vi "Measure vs B2Dv5beta_2.vi"() -> ()   [LabVIEW 2009]
doc: "This VI is an example operator panel.\n\nThe VI contains a table for the field values that may be configured manually, or loaded by checking the \"Prompt for File\" box. The data file should contain 3 columns of data, with each column delimited by a tab character.\n\nBefore the VI is executed, set the desired field units and coordinate system. Once the VI is started, follow the directions in the STATUS indicator to operate. Once a field value is achieved, it will be held indefinitely with no user intervention.\n\nThe present field is displayed in the selected units and coordinate system. The present field is queried once per second.\n\nIf a field point is specified that is outside the limits for the magnet, the VI will abort execution."
uses:
  <vilib>/Utility/file.llb/Read From Spreadsheet File (DBL).vi
panel:
  in  "AH":bool=TRUE
  in  "GPIB HP 2":string="13"
  in  "Z-Axis ramp?":bool=TRUE
  in  "Y- Axis ramp?":bool=TRUE
  out "Ist-Länge":dbl=0.009099999999997922
  out "z input":dbl=-3.5494
  out "y input":dbl=-3.5137
  out "Soll-Länge":dbl=4.994429702178218
  in  "FieldRange":dbl=1.0
  in  "Change\nPID\n(DetermineSIMPID.vi)":bool
  in  "X Axis":enum16{"B", "phi"}(ring)=enum."phi"
  in  "Y Axis":T1(ring)=enum."HP (V)"
  out "measured data":dbl[][](array[numeric])
  out "XY Graph":T2(graph)
  in  "Notes:":string="Datum: 5.09.11, Uhrzeit: 17:00, T1.5K, PID LOOP: P 0.5 I 200 D off , PID Dämpfung: P -0.5 D4.4E-5 , Laser 25°, 20mA, AOM 10mA, Sweep 0.09T/min, Winkelsweep 45-225° bei 0.5 T, VectorsM1.txt,  Winkelschritt 2°, mit ManualRamp" caption="Notizen:"
  out "Messfile Refnum":refnum<file>
  in  "Measurement File":path=path "D:/UserData/Matthias/Messungen/STO_LAOR103/110905/110905_R103_0.5T_winkelsweep_M1.txt"
  in  "Sample name:":string="R103"
  in  "HP 1":bool=TRUE
  in  "GPIB HP":string="14"
  in  "HP 2":bool=TRUE
  in  "LI 3":bool
  in  "GPIB L 3":string="8"
  in  "LI 2":bool
  in  "GPIB L 2":string="8"
  in  "LI 1":bool
  in  "GPIB L 1":string="8"
  out "Number of lines":i32=91
  out "Ramp Rate along Vector (T/min)":dbl=0.09 format="%.3f"
  out "Current Ramp Rate Z (T/min)":dbl=0.06396045575747722 format="%.3f"
  out "Current Ramp Rate Y (T/min)":dbl=0.06331713906436233 format="%.3f"
  in  "User defined Ramp Rate (T/min)":bool=TRUE
  in  "User defined Ramp Rate (T/min)":dbl=0.09 format="%.3f"
  in  "Z-Axis Communications Config":T3={"GPIB address"=22, "GPIB bus"=1, "connection ID"=refnum, "IP"="111.111.111.1", "Active Comm Interface"=0, "Serial Port"="", "Programmer Type"=0} {"Programmer Type" items=["Model 430", "Model 420"]; "Active Comm Interface" items=["TCP/IP (Model 430 Only)", "RS232", "IEEE488"]}
  in  "Max Ramp Rate - Y Axis (A/s)":dbl=0.055 format="%.3f"
  in  "Max Ramp Rate - Z Axis (A/s)":dbl=0.19 format="%.3f"
  in  "Magnitude Limit (kG)":dbl=45.1 format="%.3f"
  in  "Y-Axis Communications Config":T3={"GPIB address"=22, "GPIB bus"=1, "connection ID"=refnum, "IP"="111.111.111.2", "Active Comm Interface"=0, "Serial Port"="", "Programmer Type"=0} {"Programmer Type" items=["Model 430", "Model 420"]; "Active Comm Interface" items=["TCP/IP (Model 430 Only)", "RS232", "IEEE488"]}
  out "Cartesian Display (T)":T4={"Y-Axis Field (T)"=-8e-05, "Z-Axis Field (T)"=0.00027} {"Z-Axis Field (T)" format="%.3f"; "Y-Axis Field (T)" format="%.3f"}
  in  "Starting index":i32=92
  in  "Normal color":u32(colorbox)=11711154
  in  "Highlight color":u32(colorbox)=16711680
  in  "Prompt for File?":bool=TRUE
  out "Continue Execution?":bool=TRUE
  out "error out":T5
  in  "error in":T5
  out "STATUS":string="Zeroing vector."
  in  "Ramping Control":u16(ring)=4 items=["NEXT VECTOR", "RAMPING", "HOLDING", "PAUSE", "ZERO"]
  out "Cartesian Display (kG)":T6 {"Z-Axis Field (kG)" format="%.3f"; "Y-Axis Field (kG)" format="%.3f"}
  in  "Field Values":string[][](table)=[["0.5000", "45.0000"], ["0.5000", "47.0000"], ["0.5000", "49.0000"], ["0.5000", "51.0000"], ["0.5000", "53.0000"], ["0.5000", "55.0000"], ["0.5000", "57.0000"], ["0.5000", "59.0000"], ["0.5000", "61.0000"], ["0.5000", "63.0000"], ["0.5000", "65.0000"], ["0.5000", "67.0000"], ["0.5000", "69.0000"], ["0.5000", "71.0000"], ["0.5000", "73.0000"], ["0.5000", "75.0000"], ["0.5000", "77.0000"], ["0.5000", "79.0000"], ["0.5000", "81.0000"], ["0.5000", "83.0000"], ["0.5000", "85.0000"], ["0.5000", "87.0000"], ["0.5000", "89.0000"], ["0.5000", "91.0000"], ["0.5000", "93.0000"], ["0.5000", "95.0000"], ["0.5000", "97.0000"], ["0.5000", "99.0000"], ["0.5000", "101.0000"], ["0.5000", "103.0000"], ["0.5000", "105.0000"], ["0.5000", "107.0000"], ["0.5000", "109.0000"], ["0.5000", "111.0000"], ["0.5000", "113.0000"], ["0.5000", "115.0000"], ["0.5000", "117.0000"], ["0.5000", "119.0000"], ["0.5000", "121.0000"], ["0.5000", "123.0000"], ["0.5000", "125.0000"], ["0.5000", "127.0000"], ["0.5000", "129.0000"], ["0.5000", "131.0000"], ["0.5000", "133.0000"], ["0.5000", "135.0000"], ["0.5000", "137.0000"], ["0.5000", "139.0000"], ["0.5000", "141.0000"], ["0.5000", "143.0000"], ["0.5000", "145.0000"], ["0.5000", "147.0000"], ["0.5000", "149.0000"], ["0.5000", "151.0000"], ["0.5000", "153.0000"], ["0.5000", "155.0000"], ["0.5000", "157.0000"], ["0.5000", "159.0000"], ["0.5000", "161.0000"], ["0.5000", "163.0000"], ["0.5000", "165.0000"], ["0.5000", "167.0000"], ["0.5000", "169.0000"], ["0.5000", "171.0000"], ["0.5000", "173.0000"], ["0.5000", "175.0000"], ["0.5000", "177.0000"], ["0.5000", "179.0000"], ["0.5000", "181.0000"], ["0.5000", "183.0000"], ["0.5000", "185.0000"], ["0.5000", "187.0000"], ["0.5000", "189.0000"], ["0.5000", "191.0000"], ["0.5000", "193.0000"], ["0.5000", "195.0000"], ["0.5000", "197.0000"], ["0.5000", "199.0000"], ["0.5000", "201.0000"], ["0.5000", "203.0000"], ["0.5000", "205.0000"], ["0.5000", "207.0000"], ["0.5000", "209.0000"], ["0.5000", "211.0000"], ["0.5000", "213.0000"], ["0.5000", "215.0000"], ["0.5000", "217.0000"], ["0.5000", "219.0000"], ["0.5000", "221.0000"], ["0.5000", "223.0000"], ["0.5000", "225.0000"]]
  out "Switch Heaters":bool=TRUE
  out "Polar Display (T)":T7 {"Field Magnitude (T)" format="%.3f"; "q (degrees)" format="%.3f"}
  out "Polar Display (kG)":T8 {"Field Magnitude (kG)" format="%.3f"; "q (degrees)" format="%.3f"}
  in  "Coordinate System":u16(ring)=1 items=["Cartesian", "Polar"]
  in  "Magnetic Field Units":u16(ring)=1 items=["kG", "Tesla"]
  # "Vorsicht! Preliminary Measurement Program, watch field limits and pause the power supplies manually when stopping \nthe program!"
  # "Measurement Display"
  # "Measurement Settings"
  # "Magnet Settings"
  # "Max Ramp Rate z: 1.27 T/min\nMax Ramp Rate y: 0.17 T/min"
  # "Devices"
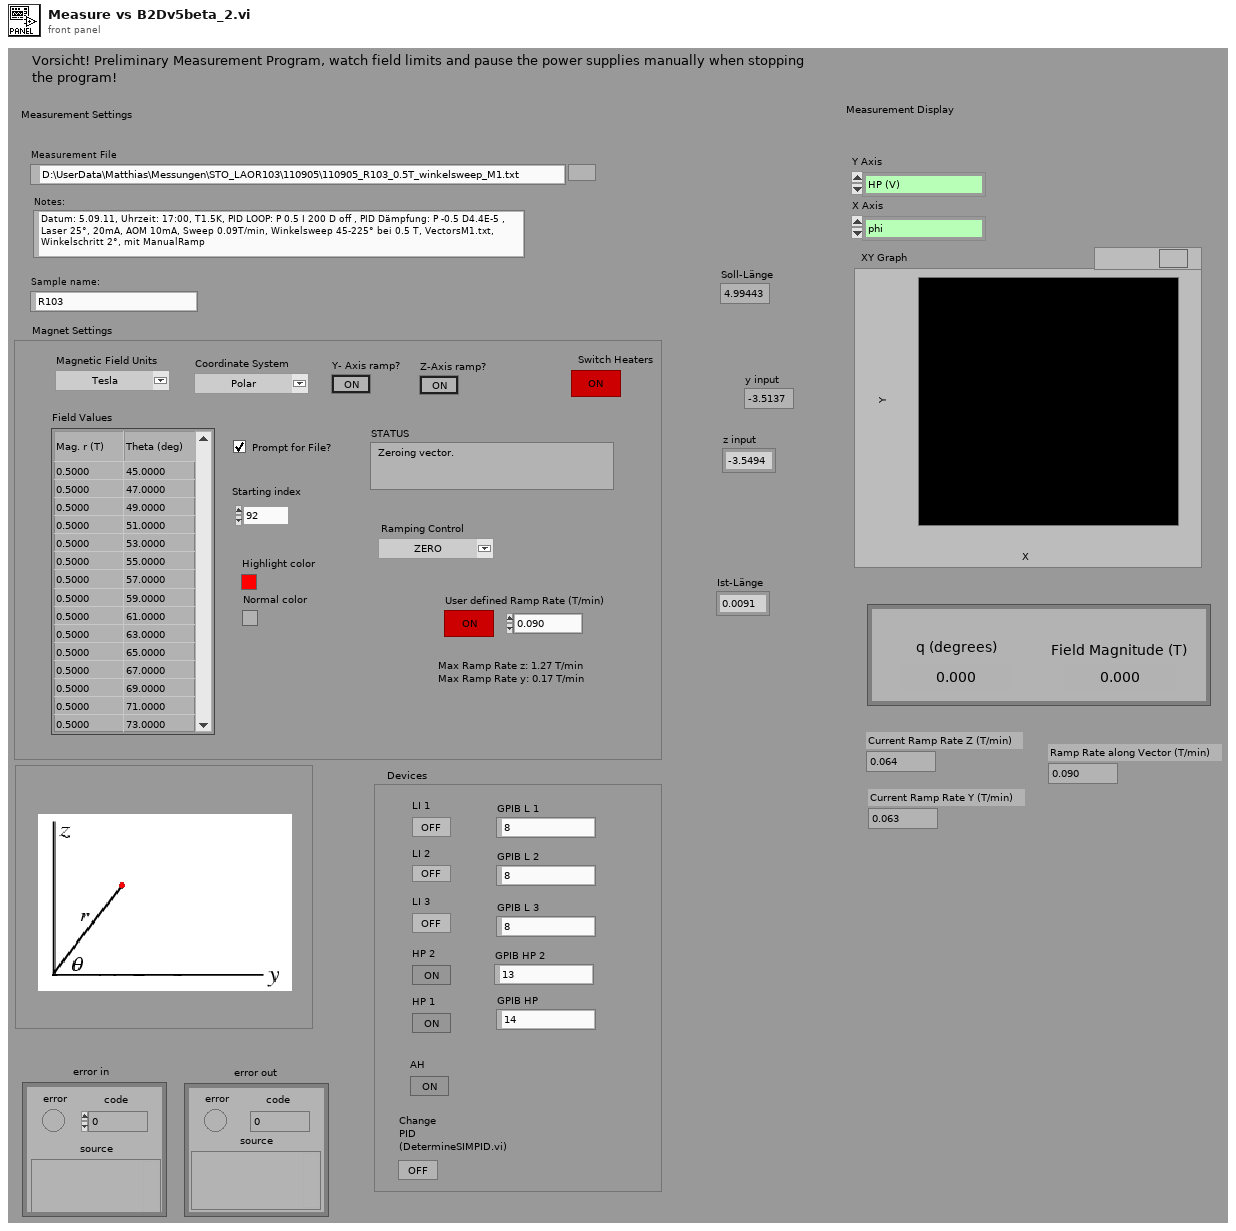
[diagram p1: front panel]
types:
  T1 = enum16{"B", "phi", "LI 1 Vx", "LI 1 phase", "LI 2 Vx", "LI 2 phase", "LI 3 Vx", "LI 3 phase", "LI 4 Vx", "LI 4 phase", "HP (V)"}
  T2 = cluster{"measured data":dbl[], "measured data":dbl[]}
  T3 = cluster{"GPIB address":i16, "GPIB bus":i16, "connection ID":refnum<k5>, "IP":string, "Active Comm Interface":u16, "Serial Port":refnum<visa-resource-name>, "Programmer Type":u16}
  T4 = cluster{"Y-Axis Field (T)":dbl, "Z-Axis Field (T)":dbl}
  T5 = cluster{"error":bool, "code":i32, "source":string}
  T6 = cluster{"Y-Axis Field (kG)":dbl, "Z-Axis Field (kG)":dbl}
  T7 = cluster{"q (degrees)":dbl, "Field Magnitude (T)":dbl}
  T8 = cluster{"q (degrees)":dbl, "Field Magnitude (kG)":dbl}
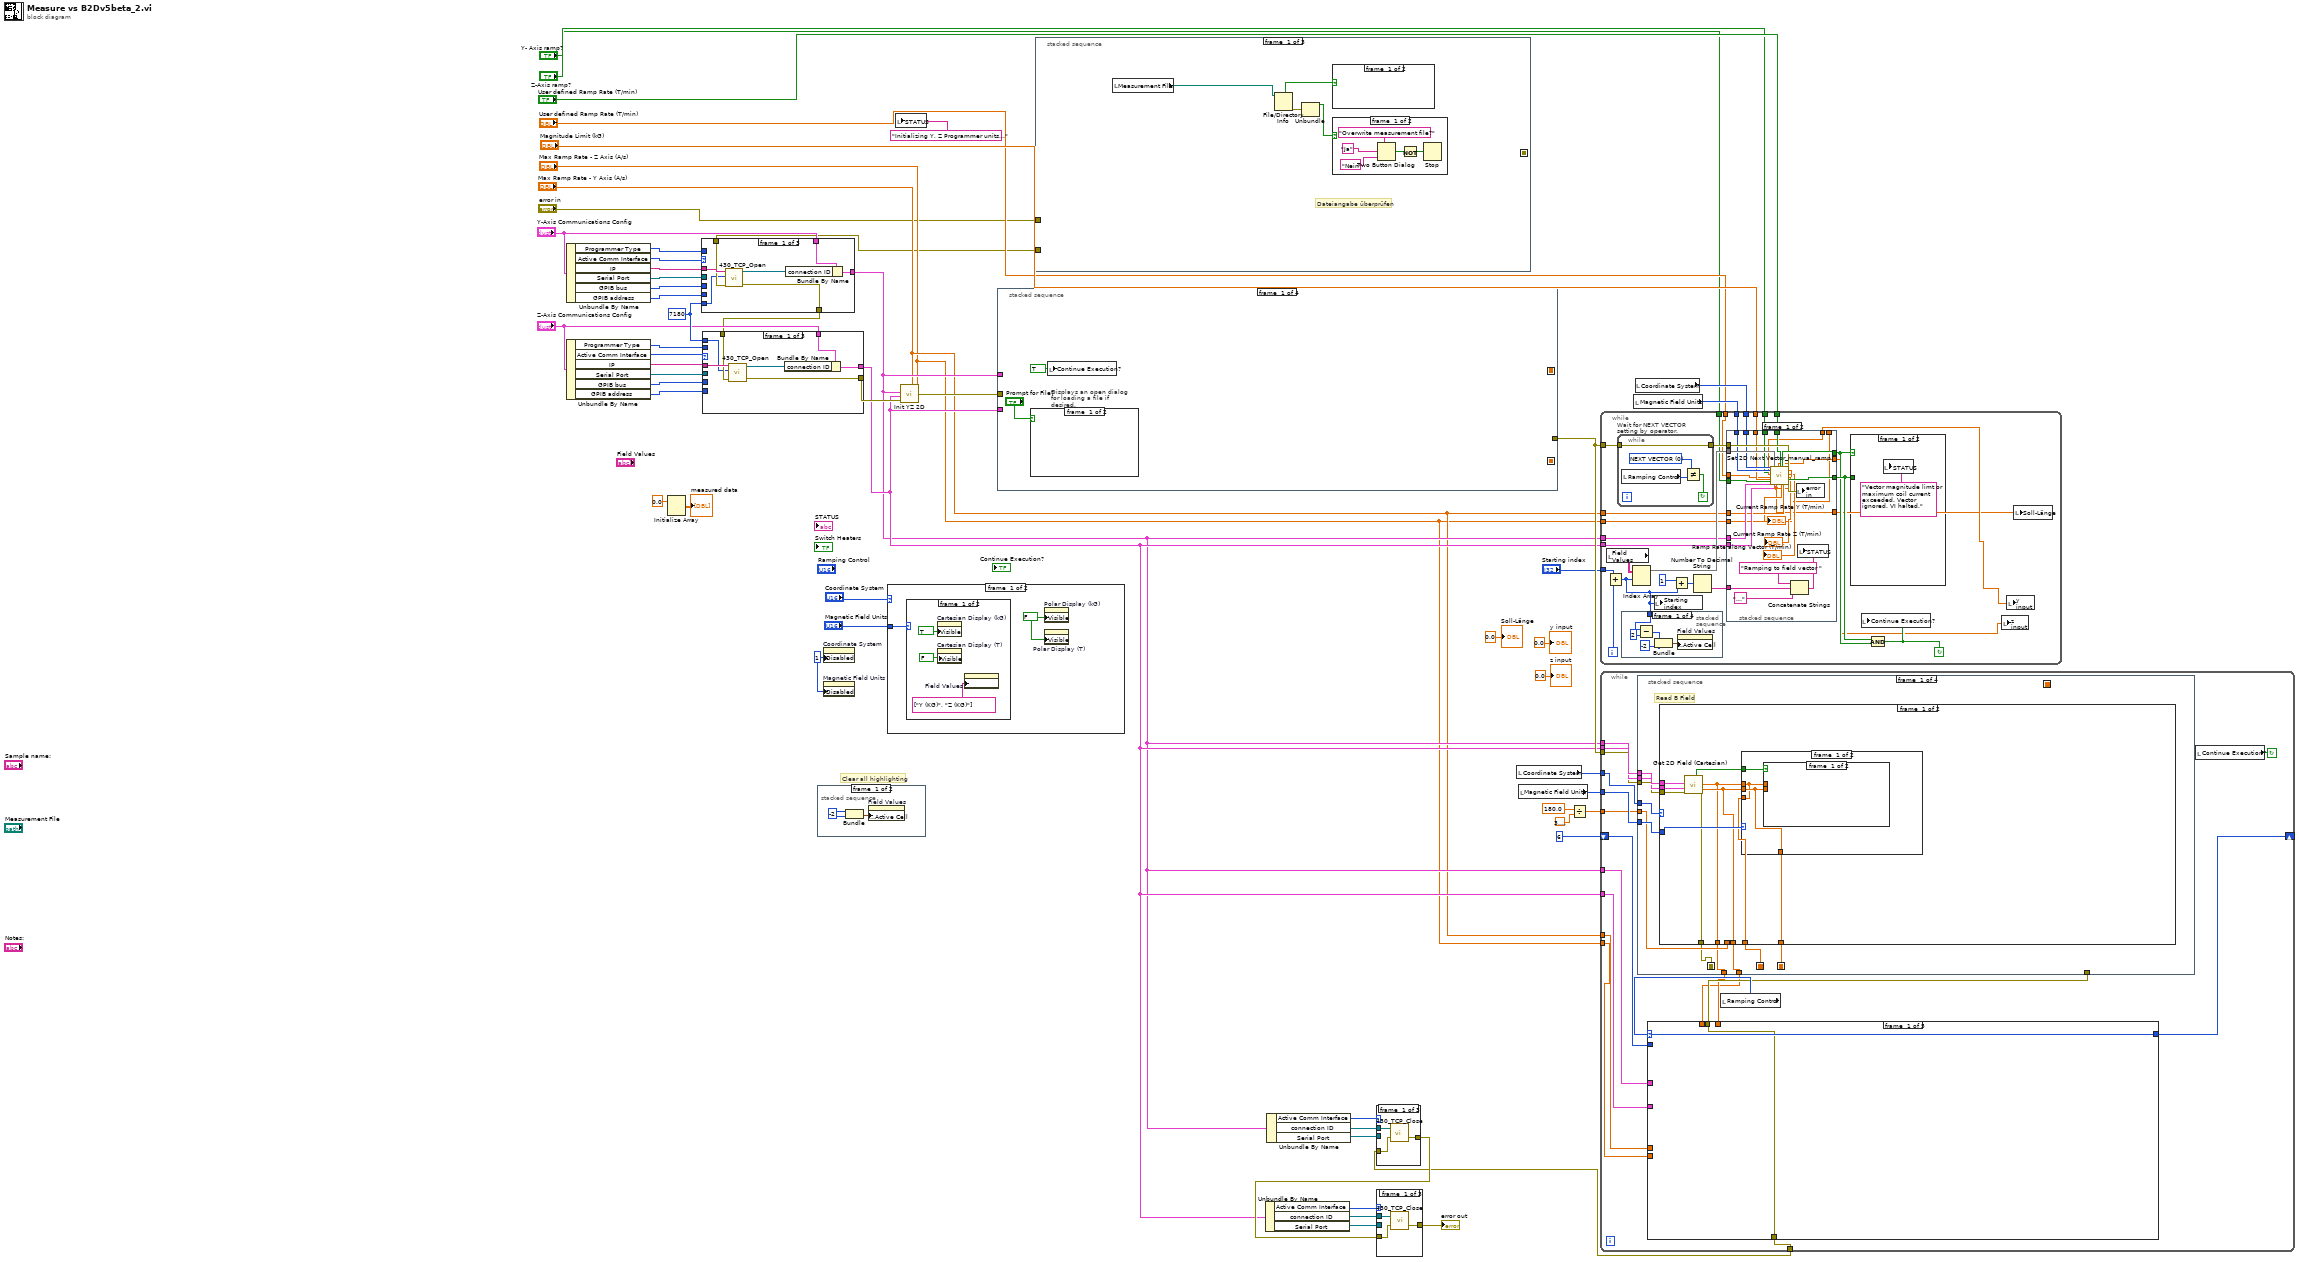
[diagram p0: block diagram]
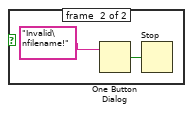
[diagram p3: hidden frame]
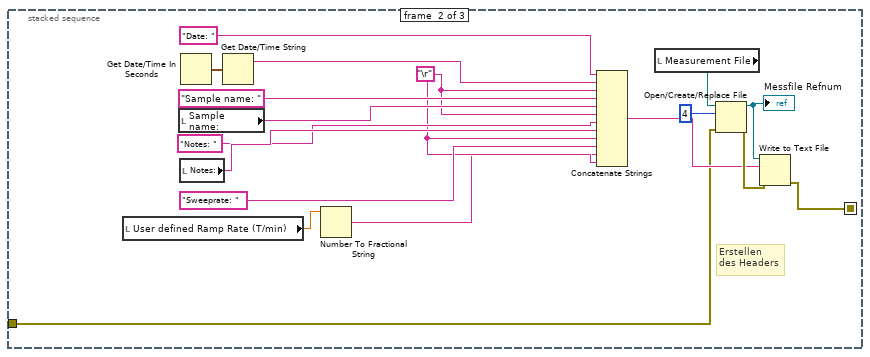
[diagram p4: hidden frame]
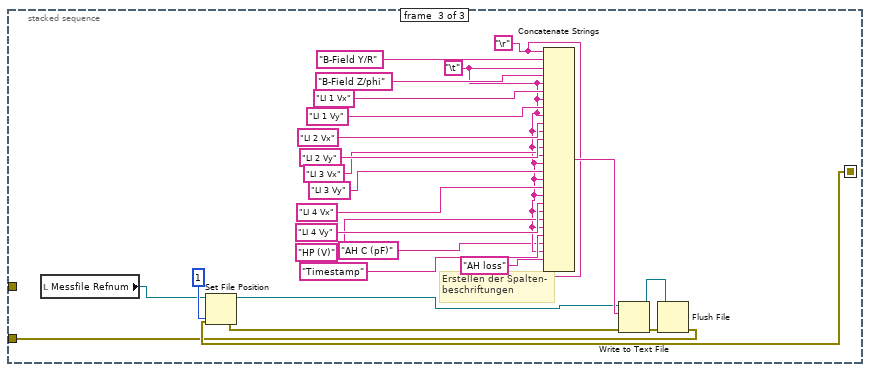
[diagram p5: hidden frame]
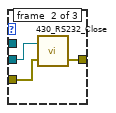
[diagram p6: hidden frame]
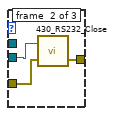
[diagram p8: hidden frame]
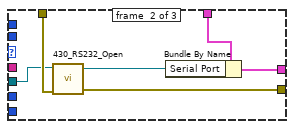
[diagram p10: hidden frame]
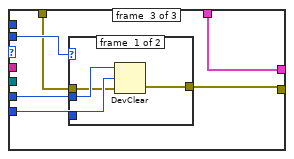
[diagram p11: hidden frame]
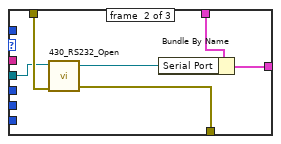
[diagram p13: hidden frame]
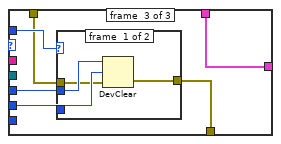
[diagram p14: hidden frame]
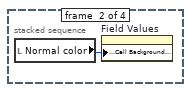
[diagram p16: hidden frame]
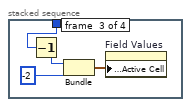
[diagram p17: hidden frame]
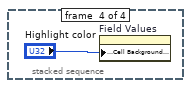
[diagram p18: hidden frame]
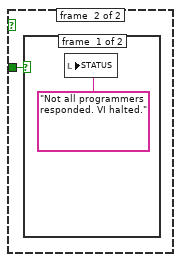
[diagram p19: hidden frame]
diagram:
  w42 = 7180 ("TCP Port")
  w55 = u8 1 ("Write Attribute")
  # "Clear all highlighting"
  n1 = Unbundle By Name("Z-Axis Communications Config") -> ("Programmer Type"=w18:u16, "Active Comm Interface"=w41:u16, "IP"=w38:string, "Serial Port"=w37:refnum<visa-resource-name>, "GPIB bus"=w17:i16, "GPIB address"=w16:i16)
  n2 = Unbundle By Name("Y-Axis Communications Config") -> ("Programmer Type"=w12:u16, "Active Comm Interface"=w40:u16, "IP"=w39:string, "Serial Port"=w36:refnum<visa-resource-name>, "GPIB bus"=w13:i16, "GPIB address"=w14:i16)
  n3 = Initialize Array(0.0 ("element")) -> (→"measured data":dbl[][])  [unwired: 2 in]
  n4 = stacked-sequence {
    frame #0 {
      w58 = -2
      n5 = Bundle(w58, w58) -> (w59:cluster{i32, i32})  [unwired: 1 in]
      n6 = property on="Field Values" class="Tbl (strict)"("Active Cell:Active Cell"=w59) -> ()  [unwired: 2 in, 2 out]
    }
    frame #1 {
      n7 = property on="Field Values" class="Tbl (strict)"("Active Cell:Cell Background Color"="Normal color") -> ()  [unwired: 2 in, 2 out]
    }
  }
  n8 = property on="Coordinate System" class="Ring (strict)"("Disabled"=w55) -> ()  [unwired: 2 in, 2 out]
  n9 = property on="Magnetic Field Units" class="Ring (strict)"("Disabled"=w55) -> ()  [unwired: 2 in, 2 out]
  n10 = case shown="0, Default" "Coordinate System" {
    tunnel: "Magnetic Field Units" -> [w62 w70]
    frame #0 {
      w61 = FALSE ("Write Attribute")
      (unwired) FALSE ("Write Attribute")
      (unwired) TRUE ("Write Attribute")
      n11 = case shown="1" w62 {
        frame #0 {
          n12 = property on="Cartesian Display (kG)" class="Cluster (strict)"("Visible"=TRUE ("Write Attribute")) -> ()  [unwired: 2 in, 2 out]
          n13 = property on="Cartesian Display (T)" class="Cluster (strict)"("Visible"=FALSE ("Write Attribute")) -> ()  [unwired: 2 in, 2 out]
          n14 = property on="Field Values" class="Tbl (strict)"("Column Header Strings[]"=string[] ["Y (KG)", "Z (KG)"] ("Write Attribute")) -> ()  [unwired: 2 in, 2 out]
        }
        frame #1 {
          n15 = property on="Cartesian Display (kG)" class="Cluster (strict)"("Visible"=FALSE ("Write Attribute")) -> ()  [unwired: 2 in, 2 out]
          n16 = property on="Cartesian Display (T)" class="Cluster (strict)"("Visible"=TRUE ("Write Attribute")) -> ()  [unwired: 2 in, 2 out]
          n17 = property on="Field Values" class="Tbl (strict)"("Column Header Strings[]"=string[] ["Y (T)", "Z (T)"] ("Write Attribute")) -> ()  [unwired: 2 in, 2 out]
        }
      }
      n18 = property on="Polar Display (kG)" class="Clust (strict)"("Visible"=w61) -> ()  [unwired: 2 in, 2 out]
      n19 = property on="Polar Display (T)" class="Clust (strict)"("Visible"=w61) -> ()  [unwired: 2 in, 2 out]
    }
    frame #1 {
      (unwired) FALSE ("Write Attribute")
      (unwired) TRUE ("Write Attribute")
      w69 = FALSE ("Write Attribute")
      n20 = case shown="1" w70 {
        frame #0 {
          n21 = property on="Polar Display (kG)" class="Clust (strict)"("Visible"=TRUE ("Write Attribute")) -> ()  [unwired: 2 in, 2 out]
          n22 = property on="Polar Display (T)" class="Clust (strict)"("Visible"=FALSE ("Write Attribute")) -> ()  [unwired: 2 in, 2 out]
          n23 = property on="Field Values" class="Tbl (strict)"("Column Header Strings[]"=string[] ["Mag. r (KG)", "Theta (deg)"] ("Write Attribute")) -> ()  [unwired: 2 in, 2 out]
        }
        frame #1 {
          n24 = property on="Polar Display (kG)" class="Clust (strict)"("Visible"=FALSE ("Write Attribute")) -> ()  [unwired: 2 in, 2 out]
          n25 = property on="Polar Display (T)" class="Clust (strict)"("Visible"=TRUE ("Write Attribute")) -> ()  [unwired: 2 in, 2 out]
          n26 = property on="Field Values" class="Tbl (strict)"("Column Header Strings[]"=string[] ["Mag. r (T)", "Theta (deg)"] ("Write Attribute")) -> ()  [unwired: 2 in, 2 out]
        }
      }
      n27 = property on="Cartesian Display (kG)" class="Cluster (strict)"("Visible"=w69) -> ()  [unwired: 2 in, 2 out]
      n28 = property on="Cartesian Display (T)" class="Cluster (strict)"("Visible"=w69) -> ()  [unwired: 2 in, 2 out]
    }
  }
  n29 = local write "STATUS"("Initializing Y, Z Programmer units..." ("STATUS")) -> ()
  n30 = stacked-sequence {
    seq-local: [_ w88 _] -> [_ _ w111]
    tunnel: "error in" -> [_ w89 _]
    tunnel: [_ _ w110] -> w8
    frame #0 {
      # "Dateiangabe überprüfen"
      n31 = local read "Measurement File"() -> (w80:path)
      n32 = File/Directory Info(path=w80) -> (directory=w78:bool, error out=w79:errorcluster)  [unwired: 1 in, 5 out]
      n33 = Unbundle(w79) -> ("status"=w77:bool)  [unwired: 2 out]
      n34 = case shown="False" w78 {
        frame #0 {
        }
        frame #1 {
          n35 = One Button Dialog(message="Invalid\nfilename!") -> (true=w86:bool)  [unwired: 1 in]
          n36 = Stop(stop? (T)=w86) -> ()
        }
      }
      n37 = case shown="False" w77 {
        frame #0 {
          n38 = Two Button Dialog(message="Overwrite measurement file?", 1:"Nein", 2:"Ja") -> (T button?=w82:bool)
          n39 = Not(x=w82) -> (.not. x?=w81:bool)
          n40 = Stop(stop? (T)=w81) -> ()
        }
        frame #1 {
        }
      }
    }
    frame #1 {
      w92 = "\r"
      # "Erstellen\ndes Headers"
      n41 = local read "User defined Ramp Rate (T/min)"() -> (w91:dbl)
      n42 = local read "Sample name:"() -> (w98:string)
      n43 = local read "Notes:"() -> (w100:string)
      n44 = Get Date/Time In Seconds() -> (seconds since 1Jan1904=w94:timestamp)
      n45 = Get Date/Time String(seconds (now)=w94) -> (date string=w96:string)  [unwired: 2 in, 1 out]
      n46 = Number To Fractional String(number=w91) -> (F-format string=w90:string)  [unwired: 3 in]
      n47 = Concatenate Strings("Date: ", w96, w92, "Sample name: ", w98, w92, "Notes: ", w100, w92, "Sweeprate: ", w90, w92) -> (w104:string)
      n48 = local read "Measurement File"() -> (w101:path)
      n49 = Open/Create/Replace File(file path (use dialog)=w101, error in=w89, operation (0:open)=4) -> (refnum out=w103:refnum<file>, error out=w105:errorcluster)  [unwired: 3 in, 1 out]
      "Messfile Refnum" <- w103
      n50 = Write to Text File(file (use dialog)=w103, text=w104, error in=w105) -> (error out=w88:errorcluster)  [unwired: 1 in, 2 out]
    }
    frame #2 {
      w108 = "\t"
      w109 = "\r"
      # "Erstellen der Spalten-\nbeschriftungen"
      n51 = local read "Messfile Refnum"() -> (w119:refnum<file>)
      n52 = Set File Position(refnum=w119, from (0:start)=1, error in=w111) -> (refnum out=w125:refnum<file>, error out=w127:errorcluster)  [unwired: 1 in]
      n53 = Concatenate Strings(w109, "B-Field Y/R", w108, "B-Field Z/phi", w108, "LI 1 Vx", w108, "LI 1 Vy", w108, "LI 2 Vx", w108, "LI 2 Vy", w108, "LI 3 Vx", w108, "LI 3 Vy", w108, "LI 4 Vx", w108, "LI 4 Vy", w108, "HP (V)", w108, "Timestamp", "AH C (pF)" ("string"), w108, "AH loss" ("string"), w109) -> (w126:string)
      n54 = Write to Text File(file (use dialog)=w125, text=w126, error in=w127) -> (refnum out=w129:refnum<file>, error out=w128:errorcluster)  [unwired: 1 in, 1 out]
      n55 = Flush File(refnum=w129, error in=w128) -> (error out=w110:errorcluster)  [unwired: 1 out]
    }
  }
  n56 = case shown="2" w40 {
    tunnel: w39 -> [w137 _ _]
    tunnel: w8 -> [w136 w143 w145]
    tunnel: "Y-Axis Communications Config" -> [w135 w138 w149]
    tunnel: [w133 w141 w149] -> w25
    tunnel: [w132 w142 w144] -> w15
    tunnel: w42 -> [w131 _ _]
    tunnel: w36 -> [_ w139 _]
    tunnel: w14 -> [_ _ w148]
    tunnel: w13 -> [_ _ w147]
    tunnel: w12 -> [_ _ w146]
    frame #0 {
      n57 = call <userlib>:"430_TCP_Open.vi"("IP Address"=w137, "TCP Port"=w131, "error in (no error)"=w136) -> ("connection ID"=w134:refnum<k5>, "error out"=w132:errorcluster)  [unwired: 3 in, 1 out]
      n58 = Bundle By Name(cluster=w135, "connection ID"=w134) -> (w133:T3)
    }
    frame #1 {
      n59 = call <userlib>:"430_RS232_Open.vi"("VISA resource name"=w139, "error in (no error)"=w143) -> ("VISA resource name out"=w140:refnum<visa-resource-name>, "error out"=w142:errorcluster)  [unwired: 5 in]
      n60 = Bundle By Name(cluster=w138, "Serial Port"=w140) -> (w141:T3)
    }
    frame #2 {
      n61 = case shown="0, Default" w146 {
        tunnel: w147 -> [w153 _]
        tunnel: w148 -> [w152 _]
        tunnel: w145 -> [w151 w154]
        tunnel: [w150 w154] -> w144
        frame #0 {
          n62 = DevClear(2:w151, 3:w152, 4:w153) -> (0:w150:errorcluster)  [unwired: 1 out]
        }
        frame #1 {
        }
      }
    }
  }
  n63 = case shown="2" w41 {
    tunnel: w38 -> [w161 _ _]
    tunnel: w15 -> [w160 w167 w169]
    tunnel: [w159 w166 w168] -> w35
    tunnel: "Z-Axis Communications Config" -> [w158 w164 w173]
    tunnel: [w156 w165 w173] -> w26
    tunnel: w42 -> [w155 _ _]
    tunnel: w37 -> [_ w162 _]
    tunnel: w18 -> [_ _ w172]
    tunnel: w17 -> [_ _ w171]
    tunnel: w16 -> [_ _ w170]
    frame #0 {
      n64 = call <userlib>:"430_TCP_Open.vi"("IP Address"=w161, "TCP Port"=w155, "error in (no error)"=w160) -> ("connection ID"=w157:refnum<k5>, "error out"=w159:errorcluster)  [unwired: 3 in, 1 out]
      n65 = Bundle By Name(cluster=w158, "connection ID"=w157) -> (w156:T3)
    }
    frame #1 {
      n66 = call <userlib>:"430_RS232_Open.vi"("VISA resource name"=w162, "error in (no error)"=w167) -> ("VISA resource name out"=w163:refnum<visa-resource-name>, "error out"=w166:errorcluster)  [unwired: 5 in]
      n67 = Bundle By Name(cluster=w164, "Serial Port"=w163) -> (w165:T3)
    }
    frame #2 {
      n68 = case shown="0, Default" w172 {
        tunnel: w171 -> [w177 _]
        tunnel: w170 -> [w176 _]
        tunnel: w169 -> [w175 w178]
        tunnel: [w174 w178] -> w168
        frame #0 {
          n69 = DevClear(2:w175, 3:w176, 4:w177) -> (0:w174:errorcluster)  [unwired: 1 out]
        }
        frame #1 {
        }
      }
    }
  }
  n70 = call <userlib>:"Init YZ 2D.vi"("Max Ramp Rate Z-axis"="Max Ramp Rate - Z Axis (A/s)", "Max Ramp Rate Y-axis"="Max Ramp Rate - Y Axis (A/s)", "error in"=w35, "Z-Axis Communications Config"=w26, "Y-Axis Communications Config"=w25) -> ("error out"=w53:T5)  [unwired: 5 in]
  n71 = stacked-sequence {
    seq-local: [_ w186 _ _] -> [_ _ w233 _]
    seq-local: [_ w185 _ _] -> [_ _ w232 _]
    tunnel: w26 -> [_ w188 _ _]
    tunnel: w53 -> [_ w189 _ _]
    tunnel: [_ w184 _ _] -> w49
    tunnel: w25 -> [_ w187 _ _]
    frame #0 {
      n72 = case "Displays an open dialog for loading a file if desired." shown="True" "Prompt for File?" {
        frame #0 {
        }
        frame #1 {
          n73 = call-poly <vilib>:"Read From Spreadsheet File.vi"() -> ("all rows"=w183:dbl[][])  [unwired: 7 in, 4 out]
          n74 = Number To Fractional String(number=w183, precision (6)=i16 4) -> (F-format string=w182:string[][])  [unwired: 2 in]
          n75 = local write "Field Values"(w182) -> ()
        }
      }
      n76 = local write "Continue Execution?"(TRUE ("Continue Execution?")) -> ()
    }
    frame #1 {
      w197 = u16 3 items=["NEXT VECTOR", "RAMPING", "HOLDING", "PAUSE", "ZERO"] ("Ramping Control")
      n77 = call <userlib>:"Get Switch Present.vi"("error in"=w189, "Communications Config"=w187) -> ("error out"=w193:T5, "Switch Present?"=w194:bool)
      n78 = case shown="True" w194 {
        tunnel: w193 -> [w215 w224]
        tunnel: w187 -> [_ w217]
        tunnel: [0.0 w221] -> w185
        tunnel: [w215 w223] -> w192
        frame #0 {
        }
        frame #1 {
          n79 = call <userlib>:"Get Switch Heater Time.vi"("error in"=w224, "Communications Config"=w217) -> ("error out"=w220:T5, "Switch Heating Time (secs)"=w222:dbl)
          n80 = call <userlib>:"Get Switch Heater.vi"("error in"=w220, "Communications Config"=w217) -> ("error out"=w219:T5, "Switch Heater Indicator"=w218:bool)
          n81 = case shown="False" w218 {
            tunnel: [w229 w230] -> w223
            tunnel: w222 -> [w227 _]
            tunnel: [w227 0.0] -> w221
            tunnel: w219 -> [w225 w230]
            tunnel: w217 -> [w226 _]
            frame #0 {
              n82 = call <userlib>:"Set Switch Heater.vi"("error in"=w225, "Switch Heater Control"=TRUE, "Communications Config"=w226) -> ("error out"=w229:T5)
            }
            frame #1 {
            }
          }
        }
      }
      n83 = call <userlib>:"Get Switch Present.vi"("error in"=w192, "Communications Config"=w188) -> ("error out"=w190:T5, "Switch Present?"=w191:bool)
      n84 = case shown="True" w191 {
        tunnel: w190 -> [w198 w207]
        tunnel: w188 -> [_ w200]
        tunnel: [0.0 w204] -> w186
        tunnel: [w198 w206] -> w184
        frame #0 {
        }
        frame #1 {
          n85 = call <userlib>:"Get Switch Heater Time.vi"("error in"=w207, "Communications Config"=w200) -> ("error out"=w203:T5, "Switch Heating Time (secs)"=w205:dbl)
          n86 = call <userlib>:"Get Switch Heater.vi"("error in"=w203, "Communications Config"=w200) -> ("error out"=w202:T5, "Switch Heater Indicator"=w201:bool)
          n87 = case shown="False" w201 {
            tunnel: [w208 w213] -> w206
            tunnel: w205 -> [w211 _]
            tunnel: [w211 0.0] -> w204
            tunnel: w202 -> [w209 w213]
            tunnel: w200 -> [w210 _]
            frame #0 {
              n88 = call <userlib>:"Set Switch Heater.vi"("error in"=w209, "Switch Heater Control"=TRUE, "Communications Config"=w210) -> ("error out"=w208:T5)
            }
            frame #1 {
            }
          }
        }
      }
      n89 = local write "Ramping Control"(w197) -> ()
      n90 = local write "Switch Heaters"(TRUE ("Switch Heater Control")) -> ()
      n91 = property on="Switch Heaters" class="Boolean (strict)"("Disabled"=u8 1 ("Write Attribute")) -> ()  [unwired: 2 in, 2 out]
    }
    frame #2 {
      n92 = Max & Min(x=w233, y=w232) -> (max(x,y)=w234:dbl)  [unwired: 1 out]
      n93 = local write "STATUS"("Heating switches..." ("STATUS")) -> ()
      n94 = Add(x=w234, y=2) -> (x+y=w238:dbl)
      n95 = property on="Ramping Control" class="Ring (strict)"("Disabled"=u8 1 ("Write Attribute")) -> ()  [unwired: 2 in, 2 out]
      n96 = Multiply(x=w238, y=1000) -> (x*y=w237:dbl)
      n97 = Wait (ms)(milliseconds to wait=w237) -> ()  [unwired: 1 out]
    }
    frame #3 {
      n98 = property on="Ramping Control" class="Ring (strict)"("Disabled"=u8 0 ("Write Attribute")) -> ()  [unwired: 2 in, 2 out]
      n99 = local write "STATUS"("Ready to ramp to first vector. Set Ramping Mode to NEXT VECTOR to begin." ("STATUS")) -> ()
      n100 = local read "Field Values"() -> (w243:string[][])
      n101 = Array Size(array=w243) -> (size(s)=w242:i32[])
      n102 = Index Array(array=w242, index=0) -> (element=→"Number of lines":i32)
    }
  }
  n103 = Unbundle By Name(w26) -> ("Active Comm Interface"=w32:u16, "connection ID"=w31:refnum<k5>, "Serial Port"=w30:refnum<visa-resource-name>)
  n104 = Unbundle By Name(w25) -> ("Active Comm Interface"=w33:u16, "connection ID"=w29:refnum<k5>, "Serial Port"=w28:refnum<visa-resource-name>)
  n105 = local read "Coordinate System"() -> (w50:u16)
  n106 = local read "Magnetic Field Units"() -> (w48:u16)
  n107 = Divide(x=180.0, y=3.141592653589793) -> (x/y=w45:dbl)
  n108 = while {
    shift-left: u16 6 ("Ramping Control") -> [w254]
    shift-right: [w255] -> _
    tunnel: [w257] -> w27
    tunnel: w26 -> [w250]
    tunnel: w25 -> [w251]
    tunnel: w45 -> [w259]
    tunnel: w48 -> [w260]
    tunnel: w49 -> [w261]
    tunnel: w26 -> [w262]
    tunnel: w25 -> [w263]
    tunnel: w50 -> [w264]
    tunnel: "Max Ramp Rate - Y Axis (A/s)" -> [w253]
    tunnel: "Max Ramp Rate - Z Axis (A/s)" -> [w252]
    stop <- w256 continue-if-true
    n109 = stacked-sequence {
      seq-local: [w269 _ _ _] -> [_ _ w377 _]
      seq-local: [w268 _ _ _] -> [_ w344 w374 _]
      seq-local: [w267 _ _ _] -> [_ _ w375 _]
      seq-local: [_ _ w361 _] -> [_ _ _ w446]
      tunnel: w264 -> [w275 _ _ w444]
      tunnel: w263 -> [w274 _ _ _]
      tunnel: w262 -> [w273 _ _ _]
      tunnel: w261 -> [w272 _ _ _]
      tunnel: w260 -> [w271 _ _ _]
      tunnel: w259 -> [w270 _ _ _]
      tunnel: [_ _ w376 _] -> w249
      tunnel: [w266 _ _ _] -> w247
      tunnel: [w265 _ _ _] -> w248
      frame #0 {
        # "Read B Field"
        n110 = case shown="0, Default" w275 {
          tunnel: w274 -> [w285 w310]
          tunnel: w273 -> [w284 w309]
          tunnel: w272 -> [w283 w308]
          tunnel: w271 -> [w282 w307]
          tunnel: w270 -> [_ w306]
          tunnel: [w280 w305] -> w269
          tunnel: [w279 w303] -> w268
          tunnel: [w278 w304] -> w267
          tunnel: [w277 w302] -> w266
          tunnel: [w276 w301] -> w265
          frame #0 {
            n111 = call <userlib>:"Get 2D Field (Cartesian).vi"("Y-Axis Communications Config"=w285, "Z-Axis Communications Config"=w284, "error in"=w283) -> ("All Instruments Responded?"=w281:bool, "Y-Axis Field (kG)"=w276:dbl, "Z-Axis Field (kG)"=w277:dbl, "error out"=w280:T5)  [unwired: 2 in]
            n112 = case shown="0, Default" w282 {
              tunnel: w276 -> [w286 w294]
              tunnel: w277 -> [w287 w295]
              tunnel: w281 -> [w288 w297]
              tunnel: [w287 w293] -> w279
              tunnel: [w286 w292] -> w278
              frame #0 {
                n113 = case shown="True" w288 {
                  tunnel: w286 -> [_ w290]
                  tunnel: w287 -> [_ w289]
                  frame #0 {
                  }
                  frame #1 {
                    n114 = Bundle("Y-Axis Field (kG)"=w290, "Z-Axis Field (kG)"=w289) -> (→"Cartesian Display (kG)":T6)  [unwired: 1 in]
                  }
                }
              }
              frame #1 {
                w296 = 0.1 ("y")
                n115 = Multiply(x=w294, y=w296) -> (x*y=w292:dbl)
                n116 = Multiply(x=w295, y=w296) -> (x*y=w293:dbl)
                n117 = case shown="True" w297 {
                  tunnel: w292 -> [_ w300]
                  tunnel: w293 -> [_ w299]
                  frame #0 {
                  }
                  frame #1 {
                    n118 = Bundle(w300, w299) -> (→"Cartesian Display (T)":cluster{dbl, dbl})  [unwired: 1 in]
                  }
                }
              }
            }
          }
          frame #1 {
            n119 = stacked-sequence {
              tunnel: w310 -> [w325]
              tunnel: w309 -> [w324]
              tunnel: w308 -> [w323]
              tunnel: w307 -> [w322]
              tunnel: w306 -> [w321]
              tunnel: [w319] -> w305
              tunnel: [w318] -> w303
              tunnel: [w317] -> w304
              tunnel: [w312] -> w302
              tunnel: [w311] -> w301
              frame #0 {
                # "Field"
                n120 = call <userlib>:"Get 2D Field (Polar).vi"("Y-Axis Communications Config"=w325, "Z-Axis Communications Config"=w324, "error in"=w323) -> ("All Instruments Responded?"=w320:bool, "Radial (r) Field (kG)"=w315:dbl, "q (radians)"=w316:dbl, "error out"=w319:T5)  [unwired: 2 in]
                n121 = Cosine(x=w316) -> (cos(x)=w313:dbl)
                n122 = Sine(x=w316) -> (sin(x)=w314:dbl)
                n123 = Compound Arithmetic op=MULTIPLY(w315, w314) -> (w312:dbl)
                n124 = case shown="1" w322 {
                  tunnel: w315 -> [w327 w339]
                  tunnel: w316 -> [w329 w338]
                  tunnel: w321 -> [w328 w337]
                  tunnel: w320 -> [w330 w336]
                  tunnel: [w327 w334] -> w318
                  tunnel: [w326 w335] -> w317
                  frame #0 {
                    n125 = Multiply(x=w329, y=w328) -> (x*y=w326:dbl)
                    n126 = case shown="True" w330 {
                      tunnel: w327 -> [_ w331]
                      tunnel: w326 -> [_ w332]
                      frame #0 {
                      }
                      frame #1 {
                        n127 = Bundle(w332, "Radial (r) Field (kG)"=w331) -> (→"Polar Display (kG)":cluster{dbl, "Radial (r) Field (kG)":dbl})  [unwired: 1 in]
                      }
                    }
                  }
                  frame #1 {
                    n128 = Multiply(x=w339, y=0.1) -> (x*y=w335:dbl)
                    n129 = Multiply(x=w338, y=w337) -> (x*y=w334:dbl)
                    n130 = case shown="True" w336 {
                      tunnel: w335 -> [_ w341]
                      tunnel: w334 -> [_ w342]
                      frame #0 {
                      }
                      frame #1 {
                        n131 = Bundle(w342, w341) -> (→"Polar Display (T)":cluster{dbl, dbl})  [unwired: 1 in]
                      }
                    }
                  }
                }
                n132 = Multiply(x=w315, y=w313) -> (x*y=w311:dbl)
              }
            }
          }
        }
      }
      frame #1 {
        # "Change PID"
        n133 = case shown="True" "Change\nPID\n(DetermineSIMPID.vi)" {
          tunnel: w344 -> [_ w349]
          frame #0 {
          }
          frame #1 {
            # "z Field Value"
            n134 = call "CheckFieldRange.vi"("Field Value"=w349) -> ("Field Range"=w346:dbl)  [unwired: 10 in]
            n135 = Equal?(x="FieldRange", y=w346) -> (x = y?=w348:bool)
            n136 = case shown="False" w348 {
              tunnel: w346 -> [w354 w355]
              frame #0 {
                n137 = local write "FieldRange"(w354) -> ()
                n138 = call "DetermineSIMPID.vi"("Field Range"=w354) -> ("D"=w352:string, "P"=w353:string)  [unwired: 7 in, 2 out]
                n139 = call "SIM960ChangeP.vi"("New D Value"=w352, "New P Value"=w353, "Port Num- PID"="1", "GPIB-Adress"="2") -> ()  [unwired: 8 in]
              }
              frame #1 {
                n140 = local write "FieldRange"(w355) -> ()
              }
            }
          }
        }
      }
      frame #2 {
        w360 = u16 2 items=["NEXT VECTOR", "RAMPING", "HOLDING", "PAUSE", "ZERO"] ("Ramping Control")
        # "Zeile in Datei schreiben"
        # "Read and Save Devices"
        n141 = stacked-sequence {
          tunnel: [w389 _ _ _ _ _ _] -> w373
          tunnel: [w388 _ _ _ _ _ _] -> w372
          tunnel: [_ w402 _ _ _ _ _] -> w369
          tunnel: [_ w400 _ _ _ _ _] -> w368
          tunnel: [_ _ w412 _ _ _ _] -> w367
          tunnel: [_ _ w411 _ _ _ _] -> w366
          tunnel: [_ _ _ w422 _ _ _] -> w365
          tunnel: [_ _ _ w422 _ _ _] -> w364
          tunnel: [_ _ _ _ w428 _ _] -> w363
          tunnel: [_ _ _ _ _ _ w440] -> w362
          tunnel: [_ _ _ _ _ w435 _] -> w357
          tunnel: [_ _ _ _ _ w434 _] -> w356
          frame #0 {
            n142 = case shown="True" "LI 1" {
              tunnel: ["0" ("Antwort2") w396] -> w391
              tunnel: ["0" ("Antwort1") w395] -> w390
              frame #0 {
              }
              frame #1 {
                n143 = call "LI-Ansteuerung.vi"("Frage2"="OUTP? 4", "Frage1"="OUTP? 1", "address string"="GPIB L 1") -> ("Antwort2"=w396:string, "Antwort1"=w395:string)
              }
            }
            n144 = Fract/Exp String To Number(string=w391) -> (number=w388:dbl)  [unwired: 3 in, 1 out]
            n145 = Fract/Exp String To Number(string=w390) -> (number=w389:dbl)  [unwired: 3 in, 1 out]
          }
          frame #1 {
            n146 = case shown="False" "LI 2" {
              tunnel: [w405 w407] -> w401
              tunnel: [w405 w406] -> w403
              frame #0 {
                w405 = "0" ("Antwort1")
              }
              frame #1 {
                n147 = call "LI-Ansteuerung.vi"("Frage2"="OUTP? 4", "Frage1"="OUTP? 1", "address string"="GPIB L 2") -> ("Antwort2"=w407:string, "Antwort1"=w406:string)
              }
            }
            n148 = Fract/Exp String To Number(string=w401) -> (number=w400:dbl)  [unwired: 3 in, 1 out]
            n149 = Fract/Exp String To Number(string=w403) -> (number=w402:dbl)  [unwired: 3 in, 1 out]
          }
          frame #2 {
            n150 = case shown="False" "LI 3" {
              tunnel: [w416 w418] -> w413
              tunnel: [w416 w417] -> w414
              frame #0 {
                w416 = "0" ("Antwort1")
              }
              frame #1 {
                n151 = call "LI-Ansteuerung.vi"("Frage2"="OUTP? 4", "Frage1"="OUTP? 1", "address string"="GPIB L 3") -> ("Antwort2"=w418:string, "Antwort1"=w417:string)
              }
            }
            n152 = Fract/Exp String To Number(string=w414) -> (number=w412:dbl)  [unwired: 3 in, 1 out]
            n153 = Fract/Exp String To Number(string=w413) -> (number=w411:dbl)  [unwired: 3 in, 1 out]
          }
          frame #3 {
            n154 = case shown="False" "HP 2" {
              tunnel: [0.0 ("Voltage") w425] -> w422
              frame #0 {
              }
              frame #1 {
                n155 = call "HP-ReadVoltagev2.vi"("String"="meas:volt:dc? 200,0.001", "HP-Mulitmeter\nGPIB Address"="GPIB HP 2") -> ("Voltage"=w425:dbl)  [unwired: 9 in]
              }
            }
          }
          frame #4 {
            n156 = case shown="True" "HP 1" {
              tunnel: [0.0 ("Voltage") w432] -> w428
              frame #0 {
              }
              frame #1 {
                n157 = call "HP-ReadVoltagev2.vi"("String"="meas:volt:dc? 200,0.001", "HP-Mulitmeter\nGPIB Address"="GPIB HP") -> ("Voltage"=w432:dbl)  [unwired: 9 in]
              }
            }
          }
          frame #5 {
            n158 = case shown="False" "AH" {
              tunnel: [w437 w439] -> w435
              tunnel: [w437 w438] -> w434
              frame #0 {
                w437 = 0.0 ("Voltage")
              }
              frame #1 {
                n159 = call "AHRead2550.vi"() -> ("loss"=w438:dbl, "capacitance"=w439:dbl)  [unwired: 9 in, 1 out]
              }
            }
          }
          frame #6 {
            n160 = Get Date/Time In Seconds() -> (seconds since 1Jan1904=w441:timestamp)
            n161 = To Double Precision Float(number=w441) -> (double precision float=w440:dbl)
          }
        }
        n162 = local read "Ramping Control"() -> (w359:u16)
        n163 = Build Array(w375, w374, w373, w372, w369, w368, w366, w367, w365, w364, w363, w362, w357, w356) -> (w361:dbl[])
        n164 = Array To Spreadsheet String(array=w361, 3:"%f" ("format string")) -> (spreadsheet string=w371:string)  [unwired: 1 in]
        n165 = Equal?(x=w359, y=w360) -> (x = y?=w358:bool)
        n166 = case shown="False" w358 {
          tunnel: w377 -> [w386 w387]
          tunnel: [w385 w387] -> w376
          tunnel: w371 -> [w384 _]
          frame #0 {
            n167 = local read "Messfile Refnum"() -> (w378:refnum<file>)
            n168 = Set File Position(refnum=w378, from (0:start)=1, error in=w386) -> (refnum out=w380:refnum<file>, error out=w381:errorcluster)  [unwired: 1 in]
            n169 = Write to Text File(file (use dialog)=w380, text=w384, error in=w381) -> (refnum out=w383:refnum<file>, error out=w382:errorcluster)  [unwired: 1 in, 1 out]
            n170 = Flush File(refnum=w383, error in=w382) -> (error out=w385:errorcluster)  [unwired: 1 out]
          }
          frame #1 {
          }
        }
      }
      frame #3 {
        n171 = local read "measured data"() -> (w447:dbl[][])
        n172 = Insert Into Array(array=w447, new element=w446) -> (w445:dbl[][])  [unwired: 2 in]
        n173 = case shown="0, Default" w444 {
          tunnel: w445 -> [w463 w477]
          tunnel: "Y Axis" -> [w465 w476]
          tunnel: "X Axis" -> [w453 w475]
          frame #0 {
            n174 = Index Array(array=w463, index (col)=1 ("disabled index (col)")) -> (element=w458:dbl[])  [unwired: 1 in]
            n175 = Index Array(array=w463, index (col)=0 ("disabled index (col)")) -> (element=w457:dbl[])  [unwired: 1 in]
            n176 = Square(x=w458) -> (x^2=w460:dbl[])
            n177 = Square(x=w457) -> (x^2=w461:dbl[])
            n178 = Index Array(array=w463, index (col)=w465) -> (element=w452:dbl[])  [unwired: 1 in]
            n179 = Divide(x=w458, y=w457) -> (x/y=w449:dbl[])
            n180 = Add(x=w461, y=w460) -> (x+y=w459:dbl[])
            n181 = Inverse Tangent(1:w449) -> (0:w448:dbl[])
            n182 = Square Root(x=w459) -> (sqrt(x)=w450:dbl[])
            n183 = Divide(x=w448, y=3.141592653589793) -> (x/y=w455:dbl[])
            n184 = Multiply(x=w455, y=180) -> (x*y=w451:dbl[])
            n185 = case shown="\"B\", Default" w453 {
              tunnel: w452 -> [w468 w471]
              tunnel: w451 -> [_ w470]
              tunnel: w450 -> [w467 _]
              frame #0 {
                n186 = Bundle(w467, "measured data"=w468) -> (w466:cluster{dbl[], "measured data":dbl[]})  [unwired: 1 in]
                n187 = local write "XY Graph"(w466) -> ()
              }
              frame #1 {
                n188 = Bundle(w470, "measured data"=w471) -> (w469:cluster{dbl[], "measured data":dbl[]})  [unwired: 1 in]
                n189 = local write "XY Graph"(w469) -> ()
              }
            }
          }
          frame #1 {
            n190 = Index Array(array=w477, index (col)=w475) -> (element=w474:dbl[])  [unwired: 1 in]
            n191 = Index Array(array=w477, index (col)=w476) -> (element=w473:dbl[])  [unwired: 1 in]
            n192 = Bundle("measured data"=w474, "measured data"=w473) -> (w472:T2)  [unwired: 1 in]
            n193 = local write "XY Graph"(w472) -> ()
          }
        }
        n194 = local write "measured data"(w445) -> ()
      }
    }
    n195 = local read "Ramping Control"() -> (w258:u16)
    n196 = case shown="4" w258 {
      selector: w258 -> [w479 w497 w525 w529 w544]
      tunnel: w251 -> [_ w481 _ w532 w549]
      tunnel: w250 -> [_ w480 _ w531 w548]
      tunnel: [w478 w493 w524 w530 w547] -> w257
      tunnel: [w479 w497 w525 w529 w544] -> w255
      tunnel: w254 -> [_ _ _ w528 w546]
      tunnel: w253 -> [_ _ _ _ w543]
      tunnel: w252 -> [_ _ _ _ w542]
      tunnel: w249 -> [w478 w487 w524 w526 w541]
      tunnel: w248 -> [_ w485 _ _ _]
      tunnel: w247 -> [_ w484 _ _ _]
      frame #0 {
      }
      frame #1 {
        n197 = local read "z input"() -> (w490:dbl)
        n198 = local read "y input"() -> (w491:dbl)
        n199 = local read "Number of lines"() -> (w496:i32)
        n200 = local read "Starting index"() -> (w495:i32)
        n201 = local read "Soll-Länge"() -> (w489:dbl)
        n202 = Less Or Equal?(x=w495, y=w496) -> (x <= y?=w494:bool)
        n203 = call "Calculate_Vector_length_brasse.vi"("Vector 2 z"=w484, "Vector 2 y"=w485, "Vector 1 z"=w490, "Vector 1 y"=w491) -> ("Length"=w492:dbl)  [unwired: 7 in]
        "Ist-Länge" <- w492
        n204 = call "Check 2D Limits_entwurf.vi"("error in"=w487, "Magnitude Limit (kG)"=45.0, "Z-Axis Communications Config"=w480, "Y-Axis Communications Config"=w481, "Z-Axis Field (kG)"=w484, "Y-Axis Field (kG)"=w485) -> ("Within Limits?"=w482:bool, "error out"=w486:T5)  [unwired: 2 in]
        n205 = Greater Or Equal?(x=w492, y=w489) -> (x >= y?=w488:bool)
        n206 = case shown="False" w482 {
          tunnel: w494 -> [_ w510]
          tunnel: [w498 w509] -> w493
          tunnel: w488 -> [_ w508]
          tunnel: w486 -> [w502 w507]
          tunnel: w481 -> [w504 w506]
          tunnel: w480 -> [w500 w505]
          frame #0 {
            w501 = u16 1 items=["RAMP", "PAUSE", "MANUAL UP", "MANUAL DOWN", "ZERO"] ("Ramping Mode")
            w503 = u16 1 items=["RAMP", "PAUSE", "MANUAL UP", "MANUAL DOWN", "ZERO"] ("Ramping Mode")
            # "Beep and pause if outside limits."
            n207 = call "Set Ramping Mode_brasse.vi"("error in"=w502, "Ramping Mode"=w503, "Communications Config"=w504) -> ("error out"=w499:T5)
            n208 = call "Set Ramping Mode_brasse.vi"("error in"=w499, "Ramping Mode"=w501, "Communications Config"=w500) -> ("error out"=w498:T5)
            n209 = call <vilib>:"Beep.vi"() -> ()  [unwired: 12 in]
          }
          frame #1 {
            n210 = case shown="False" w510 {
              tunnel: w507 -> [w514 w521]
              tunnel: [w513 w521] -> w509
              tunnel: w508 -> [_ w520]
              tunnel: w506 -> [w512 _]
              tunnel: w505 -> [w511 _]
              frame #0 {
                w517 = u16 3 items=["NEXT VECTOR", "RAMPING", "HOLDING", "PAUSE", "ZERO"] ("Ramping Control")
                w518 = u16 1 items=["RAMP", "PAUSE", "MANUAL UP", "MANUAL DOWN", "ZERO"] ("Ramping Mode")
                w519 = u16 1 items=["RAMP", "PAUSE", "MANUAL UP", "MANUAL DOWN", "ZERO"] ("Ramping Mode")
                n211 = local write "STATUS"("All Programmers are PAUSED. Set Ramping Mode to NEXT VECTOR to continue." ("STATUS")) -> ()
                n212 = local write "Ramping Control"(w517) -> ()
                n213 = call "Set Ramping Mode_brasse.vi"("error in"=w514, "Ramping Mode"=w518, "Communications Config"=w512) -> ("error out"=w515:T5)
                n214 = call "Set Ramping Mode_brasse.vi"("error in"=w515, "Ramping Mode"=w519, "Communications Config"=w511) -> ("error out"=w513:T5)
              }
              frame #1 {
                n215 = case shown="True" w520 {
                  frame #0 {
                  }
                  frame #1 {
                    n216 = stacked-sequence {
                      frame #0 {
                        w523 = u16 0 items=["NEXT VECTOR", "RAMPING", "HOLDING", "PAUSE", "ZERO"] ("Ramping Control")
                        n217 = local write "Ramping Control"(w523) -> ()
                        n218 = local write "STATUS"("Go to NEXT VECTOR" ("STATUS")) -> ()
                      }
                    }
                  }
                }
              }
            }
          }
        }
      }
      frame #2 {
      }
      frame #3 {
        n219 = Not Equal?(x=w529, y=w528) -> (x != y?=w527:bool)
        n220 = case shown="True" w527 {
          tunnel: w532 -> [_ w540]
          tunnel: w531 -> [_ w539]
          tunnel: [w533 w537] -> w530
          tunnel: w526 -> [w533 w534]
          frame #0 {
          }
          frame #1 {
            w535 = u16 1 items=["RAMP", "PAUSE", "MANUAL UP", "MANUAL DOWN", "ZERO"] ("Ramping Mode")
            # "Beep if outside limits."
            n221 = call <userlib>:"Set Ramping Mode.vi"("error in"=w534, "Ramping Mode"=w535, "Communications Config"=w540) -> ("error out"=w538:T5)
            n222 = call <userlib>:"Set Ramping Mode.vi"("error in"=w538, "Ramping Mode"=w535, "Communications Config"=w539) -> ("error out"=w537:T5)
            n223 = call <vilib>:"Beep.vi"() -> ()  [unwired: 12 in]
            n224 = local write "STATUS"("All Programmers are PAUSED. Set Ramping Mode to NEXT VECTOR to continue." ("STATUS")) -> ()
          }
        }
      }
      frame #4 {
        n225 = Not Equal?(x=w544, y=w546) -> (x != y?=w545:bool)
        n226 = case shown="True" w545 {
          tunnel: w549 -> [_ w558]
          tunnel: w548 -> [_ w557]
          tunnel: [w550 w553] -> w547
          tunnel: w543 -> [_ w556]
          tunnel: w542 -> [_ w555]
          tunnel: w541 -> [w550 w551]
          frame #0 {
          }
          frame #1 {
            w552 = u16 4 items=["RAMP", "PAUSE", "MANUAL UP", "MANUAL DOWN", "ZERO"] ("Ramping Mode")
            n227 = local write "STATUS"("Zeroing vector." ("STATUS")) -> ()
            n228 = call <userlib>:"Set Ramping Mode.vi"("error in"=w551, "Ramping Mode"=w552, "Communications Config"=w558) -> ("error out"=w561:T5)
            n229 = call <userlib>:"Set Ramping Mode.vi"("error in"=w561, "Ramping Mode"=w552, "Communications Config"=w557) -> ("error out"=w554:T5)
            n230 = call <userlib>:"Set Current Ramp Rate.vi"("Communications Config"=w558, "Ramp Rate (A/sec)"=w556, "error in"=w554) -> ("error out"=w559:T5)  [unwired: 2 in]
            n231 = call <userlib>:"Set Current Ramp Rate.vi"("Communications Config"=w557, "Ramp Rate (A/sec)"=w555, "error in"=w559) -> ("error out"=w553:T5)  [unwired: 2 in]
          }
        }
      }
    }
    n232 = local read "Continue Execution?"() -> (w256:bool)
  }
  n233 = case shown="0, Default" w33 {
    tunnel: w29 -> [w564 _ _]
    tunnel: w27 -> [w563 w567 w568]
    tunnel: [w562 w566 w568] -> w34
    tunnel: w28 -> [_ w565 _]
    frame #0 {
      n234 = call <userlib>:"430_TCP_Close.vi"("error in (no error)"=w563, "connection ID"=w564) -> ("error out"=w562:errorcluster)  [unwired: 1 out]
    }
    frame #1 {
      n235 = call <userlib>:"430_RS232_Close.vi"("error in (no error)"=w567, "VISA resource name"=w565) -> ("error out"=w566:errorcluster)  [unwired: 1 in]
    }
    frame #2 {
    }
  }
  n236 = case shown="0, Default" w32 {
    tunnel: w31 -> [w571 _ _]
    tunnel: w34 -> [w570 w574 w575]
    tunnel: [w569 w573 w575] -> w24
    tunnel: w30 -> [_ w572 _]
    frame #0 {
      n237 = call <userlib>:"430_TCP_Close.vi"("error in (no error)"=w570, "connection ID"=w571) -> ("error out"=w569:errorcluster)  [unwired: 1 out]
    }
    frame #1 {
      n238 = call <userlib>:"430_RS232_Close.vi"("error in (no error)"=w574, "VISA resource name"=w572) -> ("error out"=w573:errorcluster)  [unwired: 1 in]
    }
    frame #2 {
    }
  }
  "error out" <- w24
  n239 = local read "Magnetic Field Units"() -> (w51:u16)
  n240 = local read "Coordinate System"() -> (w52:u16)
  n241 = while {
    tunnel: "Starting index" -> [w588]
    tunnel: w26 -> [w594]
    tunnel: w25 -> [w595]
    tunnel: w51 -> [w596]
    tunnel: w52 -> [w597]
    tunnel: w49 -> [w600]
    tunnel: "Max Ramp Rate - Y Axis (A/s)" -> [w584]
    tunnel: "Max Ramp Rate - Z Axis (A/s)" -> [w583]
    tunnel: "Magnitude Limit (kG)" -> [w585]
    tunnel: "User defined Ramp Rate (T/min)" -> [w582]
    tunnel: "User defined Ramp Rate (T/min)" -> [w581]
    tunnel: "Z-Axis ramp?" -> [w577]
    tunnel: "Y- Axis ramp?" -> [w576]
    i -> [w587]
    stop <- w589 continue-if-true
    n242 = local read "Field Values"() -> (w591:string[][])
    n243 = Add(x=w588, y=w587) -> (x+y=w586:i32)
    n244 = while "Wait for NEXT VECTOR setting by operator." {
      tunnel: [w604] -> w599
      tunnel: w600 -> [w604]
      stop <- w605 continue-if-true
      w603 = u16 0 items=["NEXT VECTOR", "RAMPING", "HOLDING", "PAUSE", "ZERO"] ("Ramping Control")
      n245 = local read "Ramping Control"() -> (w606:u16)
      n246 = Not Equal?(x=w603, y=w606) -> (x != y?=w605:bool)
    }
    n247 = stacked-sequence {
      tunnel: w586 -> [w608 _ w614 _]
      frame #0 {
        (unwired) -2
        n248 = Subtract(x=w608, y=2) -> (x-y=w611:i32)
        n249 = Bundle(w611, -2) -> (w609:cluster{i32, i32})  [unwired: 1 in]
        n250 = property on="Field Values" class="Tbl (strict)"("Active Cell:Active Cell"=w609) -> ()  [unwired: 2 in, 2 out]
      }
      frame #1 {
        n251 = local read "Normal color"() -> (w612:u32)
        n252 = property on="Field Values" class="Tbl (strict)"("Active Cell:Cell Background Color"=w612) -> ()  [unwired: 2 in, 2 out]
      }
      frame #2 {
        n253 = Decrement(x=w614) -> (x-1=w613:i32)
        n254 = Bundle(w613, -2) -> (w616:cluster{i32, i32})  [unwired: 1 in]
        n255 = property on="Field Values" class="Tbl (strict)"("Active Cell:Active Cell"=w616) -> ()  [unwired: 2 in, 2 out]
      }
      frame #3 {
        n256 = property on="Field Values" class="Tbl (strict)"("Active Cell:Cell Background Color"="Highlight color") -> ()  [unwired: 2 in, 2 out]
      }
    }
    n257 = Index Array(array=w591, index (row)=w586) -> (element=w598:string[])  [unwired: 1 in]
    n258 = local write "Starting index"(w586) -> ()
    n259 = Add(x=1, y=w586) -> (x+y=w601:i32)
    n260 = Number To Decimal String(number=w601) -> (decimal integer string=w590:string)  [unwired: 1 in]
    n261 = stacked-sequence {
      tunnel: [w646 _] -> w592
      tunnel: [w645 _] -> w593
      tunnel: w599 -> [w641 _]
      tunnel: w598 -> [w640 _]
      tunnel: w597 -> [w639 _]
      tunnel: w596 -> [w638 _]
      tunnel: w595 -> [w637 _]
      tunnel: w594 -> [w636 _]
      tunnel: w590 -> [w635 _]
      tunnel: w585 -> [w633 _]
      tunnel: w584 -> [w632 _]
      tunnel: w583 -> [w627 _]
      tunnel: w582 -> [w631 _]
      tunnel: w581 -> [w630 _]
      tunnel: [w625 _] -> w579
      tunnel: [w624 _] -> w580
      tunnel: [w623 _] -> _
      tunnel: [w623 _] -> w578
      tunnel: w577 -> [w622 _]
      tunnel: w576 -> [w621 _]
      frame #0 {
        n262 = call <userlib>:"Set 2D Next Vector_manual_ramp.vi"("Coordinate System"=w639, "Magnetic Field Units"=w638, "Z-Axis ramp?"=w622, 4:"User defined Ramp Rate (T/min)"=w630, "Magnitude Limit (kG)"=w633, "Y-Axis ramp?"=w621, "Y-Axis Communications Config"=w637, "Input Vector"=w640, "Z-Axis Communications Config"=w636, 14:"User defined Ramp Rate (T/min)"=w631, "Max Ramp Rate - Y Axis (A/s)"=w632, "error in"=w641, "Max Ramp Rate - Z Axis (A/s)"=w627) -> ("Input Vector y (kG)"=w624:dbl, "Soll - Length"=w623:dbl, "Input Vector z (kG)"=w625:dbl, "Y-Axis Ramp Rate (T/min)"=→"Current Ramp Rate Y (T/min)":dbl, "Within Limits?"=w646:bool, "Ramp Rate along Vector (T/min)"=→"Ramp Rate along Vector (T/min)":dbl, "Z-Axis Ramp Rate (T/min)"=→"Current Ramp Rate Z (T/min)":dbl, "All Instruments Responded?"=w645:bool, "error out"=w634:T5)  [unwired: 6 in]
        n263 = Concatenate Strings("Ramping to field vector " ("STATUS"), w635, "..." ("STATUS")) -> (w642:string)
        n264 = local write "error in"(w634) -> ()
        n265 = local write "STATUS"(w642) -> ()
      }
      frame #1 {
        w647 = u16 1 items=["NEXT VECTOR", "RAMPING", "HOLDING", "PAUSE", "ZERO"] ("Ramping Control")
        n266 = local write "Ramping Control"(w647) -> ()
      }
    }
    n267 = case shown="False" w592 {
      tunnel: w593 -> [_ w619]
      frame #0 {
        n268 = local write "STATUS"("Vector magnitude limt or maximum coil current exceeded. Vector ignored. VI halted." ("STATUS")) -> ()
      }
      frame #1 {
        n269 = case shown="False" w619 {
          frame #0 {
            n270 = local write "STATUS"("Not all programmers responded. VI halted." ("STATUS")) -> ()
          }
          frame #1 {
          }
        }
      }
    }
    n271 = Compound Arithmetic op=AND(w593, w592) -> (w589:bool)
    n272 = local write "Continue Execution?"(w589) -> ()
    n273 = local write "z input"(w579) -> ()
    n274 = local write "y input"(w580) -> ()
    n275 = local write "Soll-Länge"(w578) -> ()
  }
  "Soll-Länge" <- 0.0 ("new Vector length")
  "y input" <- 0.0 ("new Vector length")
  "z input" <- 0.0 ("Vector length")
